vi "MFR Flow to SP 2-2.vi"(10 "MFC SPs":dbl[](array[numeric])) -> (2 "MFC array":dbl[](array[numeric]))   [LabVIEW 2014]
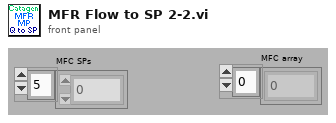
[diagram p1: front panel]
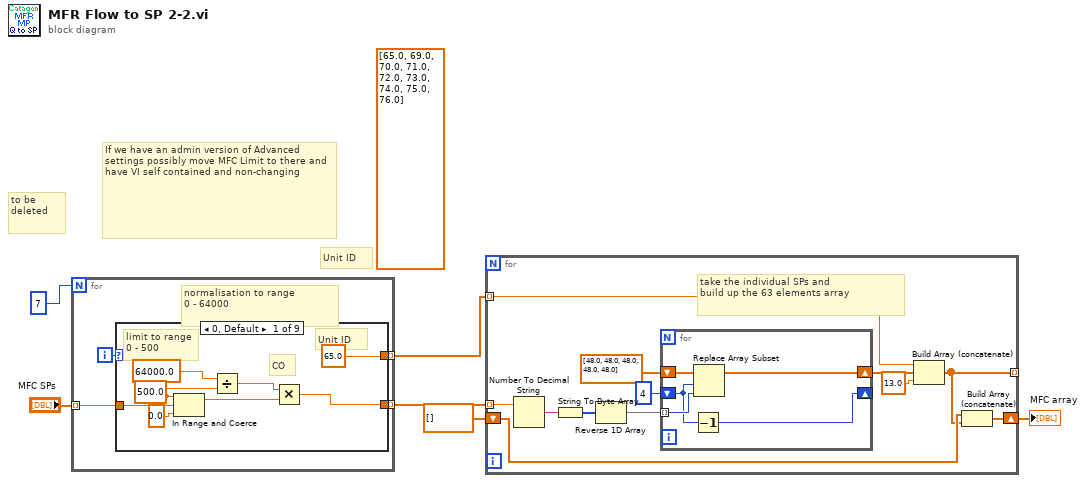
[diagram p0: block diagram]
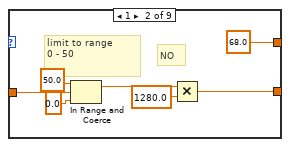
[diagram p2: hidden frame]
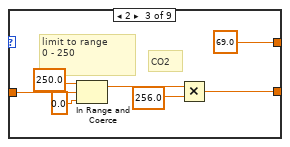
[diagram p3: hidden frame]
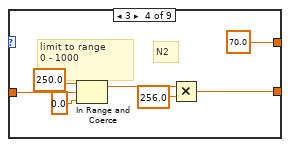
[diagram p4: hidden frame]
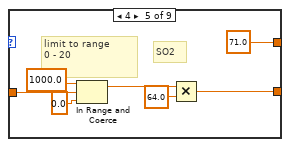
[diagram p5: hidden frame]
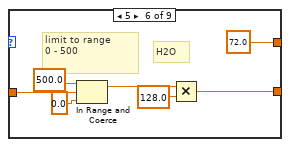
[diagram p6: hidden frame]
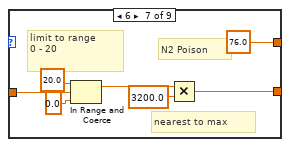
[diagram p7: hidden frame]
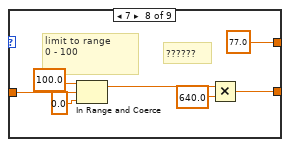
[diagram p8: hidden frame]
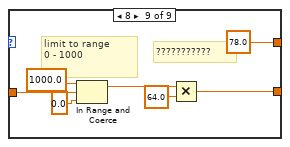
[diagram p9: hidden frame]
diagram:
  (unwired) dbl[] [65.0, 69.0, 70.0, 71.0, 72.0, 73.0, 74.0, 75.0, 76.0]
  # "to be \ndeleted"
  # "If we have an admin version of Advanced settings possibly move MFC Limit to there and have VI self contained and non-changing"
  # "Unit ID"
  n1 = for {
    N: 7 ("Numeric") -> [_]
    tunnel: "MFC SPs" -> [w9] mode=indexing
    tunnel: [w8] -> w3 mode=indexing
    tunnel: [w7] -> w2 mode=indexing
    i -> [w10]
    # "normalisation to range\n0 - 64000"
    n2 = case shown="0, Default" w10 {
      tunnel: w9 -> [w16 w21 w28 w35 w42 w49 w56 w64 w70]
      tunnel: [w18 w24 w31 w38 w45 w52 w59 w66 w73] -> w8
      tunnel: [65.0 ("y") 68.0 ("y") 69.0 ("y") 70.0 ("y") 71.0 ("y") 72.0 ("y") 76.0 ("y") 77.0 ("y") 78.0 ("y")] -> w7
      frame 0, Default {
        w14 = 500.0 ("upper limit")
        # "Unit ID"
        # "CO"
        # "limit to range\n0 - 500"
        n3 = In Range and Coerce(upper limit=w14, x=w16, lower limit=0.0) -> (coerced(x)=w13:dbl)  [unwired: 1 out]
        n4 = Divide(x=64000.0, y=w14) -> (x/y=w12:dbl)
        n5 = Multiply(x=w12, y=w13) -> (x*y=w18:dbl)
      }
      frame 1 {
        # "NO"
        # "limit to range\n0 - 50"
        n6 = In Range and Coerce(upper limit=50.0, x=w21, lower limit=0.0) -> (coerced(x)=w20:dbl)  [unwired: 1 out]
        n7 = Multiply(x=w20, y=1280.0) -> (x*y=w24:dbl)
      }
      frame 2 {
        # "CO2"
        # "limit to range\n0 - 250"
        n8 = In Range and Coerce(upper limit=250.0, x=w28, lower limit=0.0) -> (coerced(x)=w27:dbl)  [unwired: 1 out]
        n9 = Multiply(x=w27, y=256.0) -> (x*y=w31:dbl)
      }
      frame 3 {
        # "N2"
        # "limit to range\n0 - 1000"
        n10 = In Range and Coerce(upper limit=250.0, x=w35, lower limit=0.0) -> (coerced(x)=w34:dbl)  [unwired: 1 out]
        n11 = Multiply(x=w34, y=256.0) -> (x*y=w38:dbl)
      }
      frame 4 {
        # "SO2"
        # "limit to range\n0 - 20"
        n12 = In Range and Coerce(upper limit=1000.0, x=w42, lower limit=0.0) -> (coerced(x)=w41:dbl)  [unwired: 1 out]
        n13 = Multiply(x=w41, y=64.0) -> (x*y=w45:dbl)
      }
      frame 5 {
        # "H2O"
        # "limit to range\n0 - 500"
        n14 = In Range and Coerce(upper limit=500.0, x=w49, lower limit=0.0) -> (coerced(x)=w48:dbl)  [unwired: 1 out]
        n15 = Multiply(x=w48, y=128.0) -> (x*y=w52:dbl)
      }
      frame 6 {
        # "nearest to max"
        # "N2 Poison"
        # "limit to range\n0 - 20"
        n16 = In Range and Coerce(upper limit=20.0, x=w56, lower limit=0.0) -> (coerced(x)=w55:dbl)  [unwired: 1 out]
        n17 = Multiply(x=w55, y=3200.0) -> (x*y=w59:dbl)
      }
      frame 7 {
        # "??????"
        # "limit to range\n0 - 100"
        n18 = In Range and Coerce(upper limit=100.0, x=w64, lower limit=0.0) -> (coerced(x)=w62:dbl)  [unwired: 1 out]
        n19 = Multiply(x=w62, y=640.0) -> (x*y=w66:dbl)
      }
      frame 8 {
        # "???????????"
        # "limit to range\n0 - 1000"
        n20 = In Range and Coerce(upper limit=1000.0, x=w70, lower limit=0.0) -> (coerced(x)=w69:dbl)  [unwired: 1 out]
        n21 = Multiply(x=w69, y=64.0) -> (x*y=w73:dbl)
      }
    }
  }
  n22 = for {
    tunnel: w2 -> [w81] mode=indexing
    tunnel: [w77] -> _ mode=indexing
    shift-right: [w76] -> w5
    shift-left: dbl[] [] -> [w78]
    tunnel: w3 -> [w75] mode=indexing
    # "take the individual SPs and \nbuild up the 63 elements array"
    n23 = Number To Decimal String(number=w75) -> (decimal integer string=w82:string)  [unwired: 1 in]
    n24 = String To Byte Array(string=w82) -> (unsigned byte array=w85:u8[])
    n25 = Reverse 1D Array(array=w85) -> (reversed array=w86:u8[])
    n26 = for {
      tunnel: w86 -> [w89] mode=indexing
      shift-right: [w88] -> _
      shift-left: u8 4 -> [w87]
      shift-right: [w90] -> w79
      shift-left: dbl[] [48.0, 48.0, 48.0, 48.0, 48.0] -> [w91]
      n27 = Decrement(x=w87) -> (x-1=w88:u8)
      n28 = Replace Array Subset(array=w91, new element=w89, index=w87) -> (w90:dbl[])
    }
    n29 = Build Array (concatenate)(w81, w79, 13.0) -> (w77:dbl[])
    n30 = Build Array (concatenate)(w78, w77) -> (w76:dbl[])
  }
  "MFC array" <- w5
